vi "15.1.1 FindPattern.vi"() -> ()   [LabVIEW 2018]
uses:
  <vilib>/vision/Image Controls.llb/IMAQ Image.ctl
  <vilib>/vision/Image Controls.llb/Vision Info Type2.ctl
  <vilib>/vision/NI_Vision_Development_Module.lvlib
panel:
  out "Image Out":T1
  out "Elapsed time (ms)":u32
  out "Matches (pixel)":T2(array[cluster]) {"Bounding Box"."y" format="%.2f"; "Bounding Box"."x" format="%.2f"; "Position"."y" format="%.2f"; "Position"."x" format="%.2f"; "Score" format="%.2f"; "Scale" format="%.2f"; "Angle" format="%.2f"}
  out "error out":errorcluster
  out "Number of Matches":i32
  in  "Template":T1
  out "Coordinate System (duplicate)":T3 {"Measurement System"."Axis Reference" items=["Direct", "Indirect"]; "Measurement System"."Angle (deg)" format="%.2f"; "Measurement System"."Origin"."Y" format="%.2f"; "Measurement System"."Origin"."X" format="%.2f"; "Reference System"."Axis Reference" items=["Direct", "Indirect"]; "Reference System"."Angle (deg)" format="%.2f"; "Reference System"."Origin"."Y" format="%.2f"; "Reference System"."Origin"."X" format="%.2f"}
  in  "Coordinate System":T3 {"Measurement System"."Axis Reference" items=["Direct", "Indirect"]; "Measurement System"."Angle (deg)" format="%.2f"; "Measurement System"."Origin"."Y" format="%.2f"; "Measurement System"."Origin"."X" format="%.2f"; "Reference System"."Axis Reference" items=["Direct", "Indirect"]; "Reference System"."Angle (deg)" format="%.2f"; "Reference System"."Origin"."Y" format="%.2f"; "Reference System"."Origin"."X" format="%.2f"}
  out "Matches (real-world)":T2(array[cluster]) {"Bounding Box"."y" format="%.2f"; "Bounding Box"."x" format="%.2f"; "Position"."y" format="%.2f"; "Position"."x" format="%.2f"; "Score" format="%.2f"; "Scale" format="%.2f"; "Angle" format="%.2f"}
  in  "error in":errorcluster
  in  "Settings":T4={"Algorithm"=2, "Number of Matches Requested"=1, "Minimum Match Score"=800.0, "SubPixel Accuracy"=TRUE, "Rotation Angle Ranges"=[], "Show Search Area"=FALSE, "Show Result"=TRUE} {"Rotation Angle Ranges"."End" format="%.1f"; "Rotation Angle Ranges"."Start" format="%.1f"; "Minimum Match Score" min=0 max=1000 format="%.2f"; "Number of Matches Requested" min=1; "Algorithm" items=["All", "Low Discrepancy Sampling", "Grayscale Value Pyramid", "Gradients Pyramid"]}
  in  "Search Rect":T5={"Left"=0, "Top"=0, "Right"=2147483647, "Bottom"=2147483647, "Rotation"=0.0} {"Rotation" format="%.2f"; "Left" scale=0.0..1024.0; "Right" scale=0.0..1024.0}
  in  "Image":T1
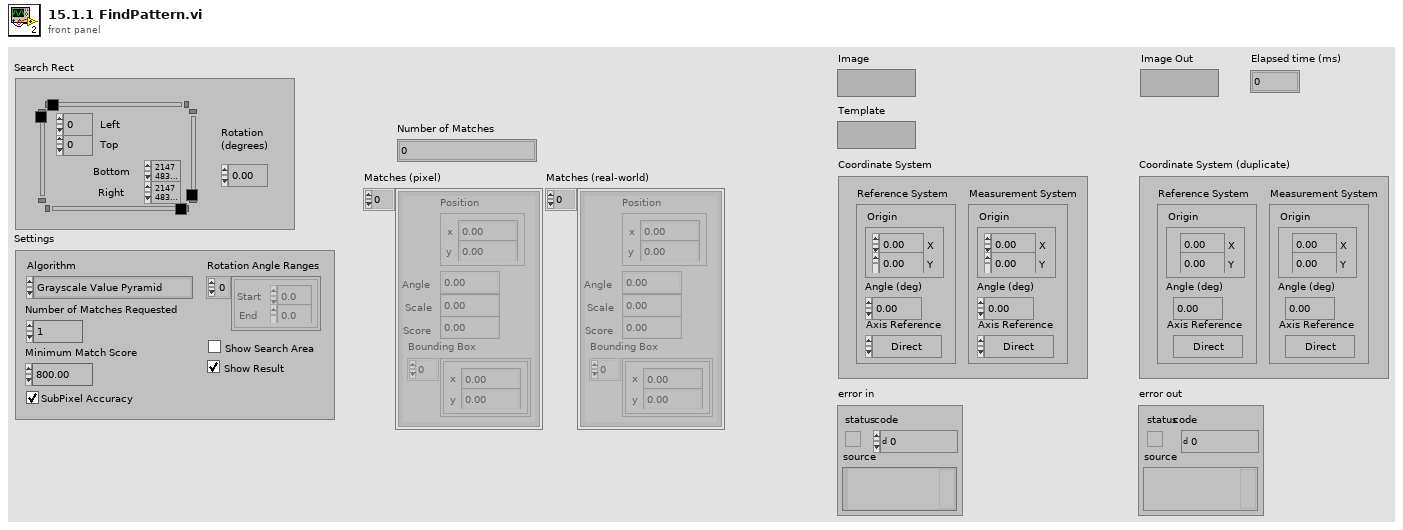
[diagram p1: front panel]
types:
  T1 = typedef "IMAQ Image.ctl" = refnum<image>
  T2 = cluster{"Position":cluster{"x":sgl, "y":sgl}, "Angle":sgl, "Scale":sgl, "Score":sgl, "Bounding Box":cluster{"x":sgl, "y":sgl}[]}[]
  T3 = typedef "IMAQ Coordinate System" = cluster{"Reference System":cluster{"Origin":cluster{"X":sgl, "Y":sgl}, "Angle (deg)":sgl, "Axis Reference":u32}, "Measurement System":cluster{"Origin":cluster{"X":sgl, "Y":sgl}, "Angle (deg)":sgl, "Axis Reference":u32}}
  T4 = cluster{"Algorithm":i32, "Number of Matches Requested":i32, "Minimum Match Score":sgl, "SubPixel Accuracy":bool, "Rotation Angle Ranges":cluster{"Start":sgl, "End":sgl}[], "Show Search Area":bool, "Show Result":bool}
  T5 = typedef "IMAQ Rectangle" = cluster{"Left":i32, "Top":i32, "Right":i32, "Bottom":i32, "Rotation":dbl}
  T6 = typedef "Vision Info Type2.ctl" = u32
  T7 = cluster{"Number of Matches Requested":i32, "Minimum Match Score":sgl, "Rotation Angle Ranges":cluster{"Start":sgl, "End":sgl}[]}
  T8 = cluster{"Show Search Area":bool, "Show Result":bool}
  T9 = cluster{"Origin":cluster{"X":sgl, "Y":sgl}, "Angle (deg)":sgl, "Axis Reference":u32}
  T10 = typedef "ROI Descriptor" = cluster{"Global Rectangle":i32[], "Contours":cluster{"ID":enum32{"External", "Internal"}, "Type":u32, "Coordinates":i32[]}[]}
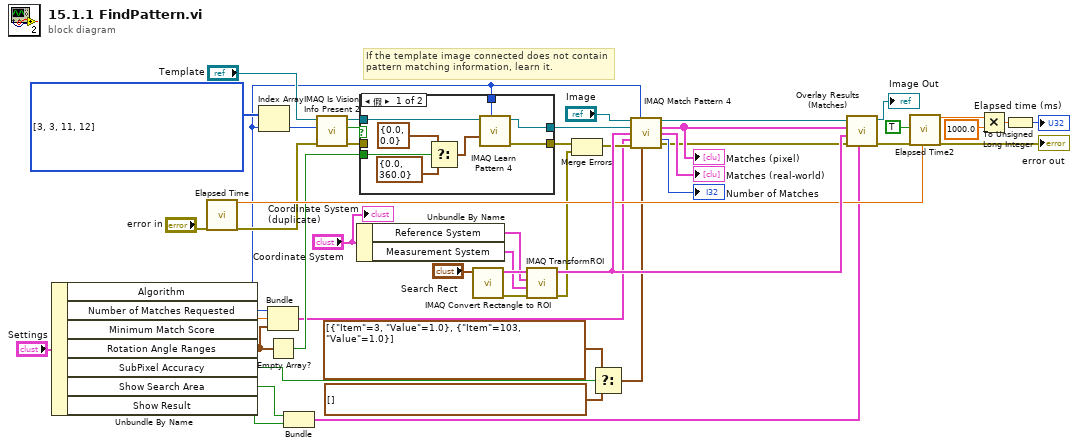
[diagram p0: block diagram]
diagram:
  w28 = T6[] [3, 3, 11, 12] items=["Any", "Calibration", "Overlay", "Grayscale Template", "Color Template", "Geometric Template", "Custom Data", "Golden Template", "Geometric Template 2", "Contour Data", "Camera Model", "Pyramid Grayvalue Template", "Pyramid Gradient Template"]
  # "If the template image connected does not contain pattern matching information, learn it."
  n1 = Unbundle By Name("Settings") -> ("Algorithm"=w4:i32, "Number of Matches Requested"=w34:i32, "Minimum Match Score"=w33:sgl, "Rotation Angle Ranges"=w8:cluster{"Start":sgl, "End":sgl}[], "SubPixel Accuracy"=w7:bool, "Show Search Area"=w6:bool, "Show Result"=w5:bool)
  n2 = call "Elapsed Time"("error in (no error)"="error in") -> ("Present (s)"=w22:dbl, "error out"=w16:errorcluster)  [unwired: 4 in, 13 out]
  n3 = Index Array(array=w28, index=w4) -> (element=w27:T6)
  n4 = Bundle("Number of Matches Requested"=w34, "Minimum Match Score"=w33, "Rotation Angle Ranges"=w8) -> (w9:T7)  [unwired: 1 out]
  n5 = Empty Array?(array=w8) -> (empty?=w11:bool)
  n6 = Bundle("Show Search Area"=w6, "Show Result"=w5) -> (w10:T8)  [unwired: 1 out]
  n7 = call "IMAQ Is Vision Info Present 2"("error in (no error)"=w16, "Vision Info"=w27, "Image"="Template") -> ("error out"=w40:errorcluster, "Present?"=w36:bool, "Image (duplicate)"=w41:T1)  [unwired: 6 out]
  n8 = Unbundle By Name("Coordinate System") -> ("Reference System"=w44:T9, "Measurement System"=w43:T9)
  n9 = case shown="假" w36 {
    tunnel: w41 -> [w52 w58]
    tunnel: w40 -> [_ w57]
    tunnel: [w56 w58] -> w37
    tunnel: [w55 w57] -> w3
    tunnel: w11 -> [w50 _]
    tunnel: w4 -> [w49 _]
    frame False {
      n10 = Select(t=cluster{"Start Angle":sgl, "End Angle":sgl} {"Start Angle"=0.0, "End Angle"=0.0} ("Angle Range"), s=w50, f=cluster{"Start Angle":sgl, "End Angle":sgl} {"Start Angle"=0.0, "End Angle"=360.0} ("Angle Range")) -> (s? t:f=w51:cluster{"Start Angle":sgl, "End Angle":sgl})
      n11 = call "IMAQ Learn Pattern 4"("Algorithm"=w49, "Angle Range"=w51, "Image"=w52) -> ("error out"=w55:errorcluster, "Template Image Out"=w56:T1)  [unwired: 3 in, 4 out]
    }
    frame True {
    }
  }
  n12 = call "IMAQ Convert Rectangle to ROI"("Rectangle"="Search Rect") -> ("error out"=w1:errorcluster, "ROI Descriptor"=w46:T10)  [unwired: 1 in, 7 out]
  n13 = call "IMAQ TransformROI"("error in (no error)"=w1, "New Reference"=w43, "Base Reference"=w44, "ROI Descriptor"=w46) -> ("error out"=w2:errorcluster, "ROI Descriptor out"=w47:T10)  [unwired: 6 out]
  n14 = Merge Errors(w3, w2) -> (w18:errorcluster)
  n15 = Select(t=cluster{"Item":u16, "Value":dbl}[] [{"Item"=3, "Value"=1.0}, {"Item"=103, "Value"=1.0}] ("Advanced Options"), s=w7, f=cluster{"Item":u16, "Value":dbl}[] [] ("Advanced Options")) -> (s? t:f=w19:cluster{"Item":u16, "Value":dbl}[])
  n16 = call "IMAQ Match Pattern 4"("Image"="Image", "Algorithm"=w4, "Template Image"=w37, "ROI Descriptor"=w47, "Parameters"=w9, "error in (no error)"=w18, "Advanced Options"=w19) -> ("Image (duplicate)"=w30:T1, "Matches (pixel)"=w31:T2, "Matches (real-world)"=→"Matches (real-world)":T2, "Number of Matches"=→"Number of Matches":i32, "error out"=w15:errorcluster)  [unwired: 1 in, 3 out]
  "Matches (pixel)" <- w31
  n17 = call "Overlay Results (Matches).vi"("Setup"=w10, "error in"=w15, "Search Area"=w47, "Matches"=w31, "Image In"=w30) -> ("error out"=w14:errorcluster, "Image Out"=→"Image Out":T1)  [unwired: 1 in, 4 out]
  n18 = call "Elapsed Time2"("Reset"=TRUE, "error in (no error)"=w14, "Set Start Time (s)"=w22) -> ("Elapsed Time (s)"=w25:dbl, "error out"=→"error out":errorcluster)  [unwired: 2 in, 13 out]
  n19 = Multiply(x=w25, y=1000.0) -> (x*y=w23:dbl)
  n20 = To Unsigned Long Integer(number=w23) -> (unsigned 32bit integer=→"Elapsed time (ms)":u32)
  "Coordinate System (duplicate)" <- "Coordinate System"
